vi "PQexecuteCommand.vi"(0 "conn":u64, 5 "Command":string, 11 "error in (no error)":errorcluster) -> (4 "conn_out":u64, 6 "Data":string[][](array[string]), 8 "ColumnNames":string[](array[string]), 10 "ColsCount":i64, 13 "error out":errorcluster, 14 "DatabaseMesssageCluster":T1, 15 "RowsCount":i64)   [LabVIEW 2019, in "libpqutility64.lvlib"]
doc: "Send arbitrari SQL command against PostgreSQL database, and fetch the result data into string array.\nSee PostgreSQL c-lib doku for further information."
uses:
  libpqutility64.lvlib
  libpqlv64/libpqlv64.lvlib
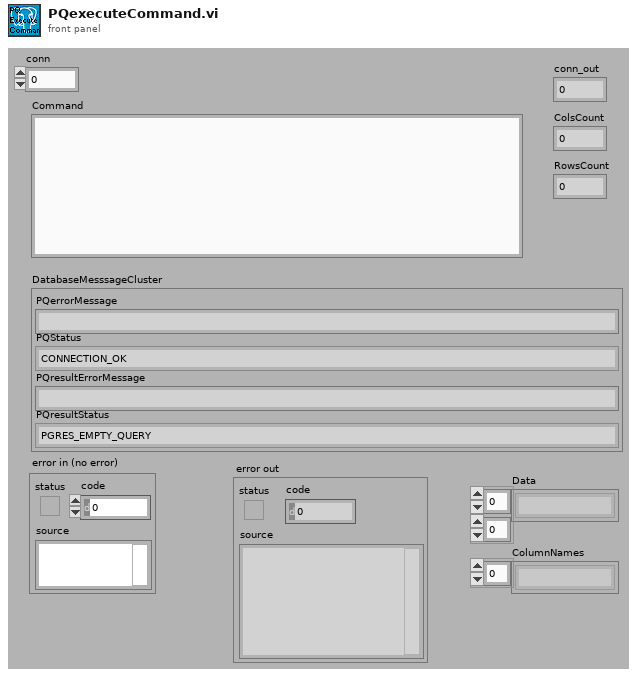
[diagram p1: front panel]
types:
  T1 = cluster{"PQerrorMessage":string, "PQStatus":enum16{"CONNECTION_OK", "CONNECTION_BAD", "CONNECTION_STARTED", "CONNECTION_MADE", "CONNECTION_AWAITING_RESPONSE", "CONNECTION_AUTH_OK", "CONNECTION_SETENV", "CONNECTION_SSL_STARTUP", "CONNECTION_NEEDED"}, "PQresultErrorMessage":string, "PQresultStatus":enum16{"PGRES_EMPTY_QUERY", "PGRES_COMMAND_OK", "PGRES_TUPLES_OK", "PGRES_COPY_OUT", "PGRES_COPY_IN", "PGRES_BAD_RESPONSE", "PGRES_NONFATAL_ERROR", "PGRES_FATAL_ERROR"}}
  T2 = enum16{"PGRES_EMPTY_QUERY", "PGRES_COMMAND_OK", "PGRES_TUPLES_OK", "PGRES_COPY_OUT", "PGRES_COPY_IN", "PGRES_BAD_RESPONSE", "PGRES_NONFATAL_ERROR", "PGRES_FATAL_ERROR"}
  T3 = enum32{"PGRES_EMPTY_QUERY", "PGRES_COMMAND_OK", "PGRES_TUPLES_OK", "PGRES_COPY_OUT", "PGRES_COPY_IN", "PGRES_BAD_RESPONSE", "PGRES_NONFATAL_ERROR", "PGRES_FATAL_ERROR"}
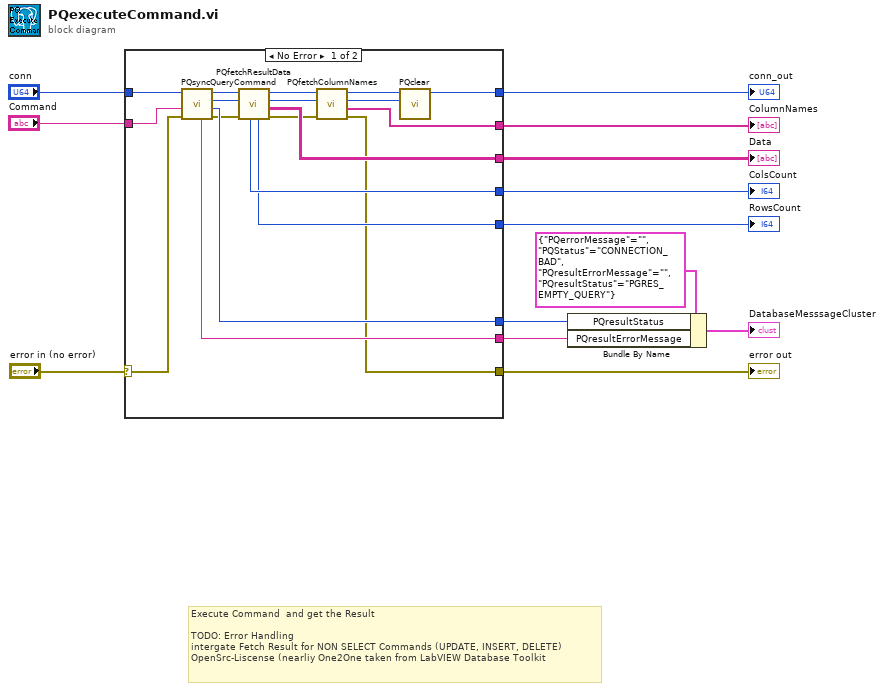
[diagram p0: block diagram]
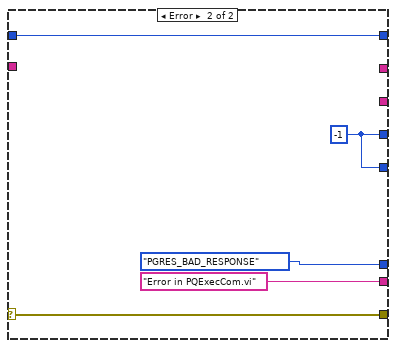
[diagram p2: hidden frame]
diagram:
  # "Execute Command  and get the Result\n\nTODO: Error Handling\nintergate Fetch Result for NON SELECT Commands (UPDATE, INSERT, DELETE)\nOpenSrc-Liscense (nearliy One2One taken from LabVIEW Database Toolkit"
  n1 = case shown="No Error" "error in (no error)" {
    selector: "error in (no error)" -> [w17 w33]
    tunnel: [w14 w33] -> w9
    tunnel: "conn" -> [w32 w37]
    tunnel: [w28 _] -> w13
    tunnel: [w29 w37] -> w2
    tunnel: [w23 _] -> w12
    tunnel: [w22 w36] -> w11
    tunnel: [w21 w36] -> w10
    tunnel: "Command" -> [w20 _]
    tunnel: [w19 T2."PGRES_BAD_RESPONSE" ("PQresultStatus")] -> w6
    tunnel: [w18 "Error in PQExecCom.vi" ("PQresultErrorMessage")] -> w5
    frame No Error {
      n2 = call "PQsyncQueryCommand.vi"("error in (no error)"=w17, "query"=w20, "conn"=w32) -> ("error out"=w16:errorcluster, "PQresultStatus"=w19:T3, "PGresult"=w31:u64, "conn out"=w30:u64, "PQresultErrorMessage"=w18:string)  [unwired: 4 in]
      n3 = call "PQfetchResultData.vi"("error in"=w16, "res"=w31, "conn"=w30) -> ("error out"=w15:errorcluster, "Data"=w28:string[][], "res_out"=w27:u64, "conn_out"=w26:u64, "PQnFields"=w21:i64, "PQnTuples"=w22:i64)  [unwired: 3 in]
      n4 = call "PQfetchColumnNames.vi"("error in"=w15, "res"=w27, "conn"=w26) -> ("error out"=w14:errorcluster, "ColumnNames"=w23:string[], "res_out"=w24:u64, "conn_out"=w25:u64)  [unwired: 3 in]
      n5 = call "PQclear.vi"("res"=w24, "conn"=w25) -> ("conn_out"=w29:u64)  [unwired: 8 in, 1 out]
    }
    frame Error {
      w36 = i64 -1 ("PQnFields")
    }
  }
  "error out" <- w9
  "Data" <- w13
  "conn_out" <- w2
  "ColumnNames" <- w12
  "ColsCount" <- w11
  "RowsCount" <- w10
  n6 = Bundle By Name(cluster=T1 {"PQerrorMessage"="", "PQStatus"=enum."CONNECTION_BAD", "PQresultErrorMessage"="", "PQresultStatus"=enum."PGRES_EMPTY_QUERY"} ("Database Status Message 2"), "PQresultStatus"=w6, "PQresultErrorMessage"=w5) -> (→"DatabaseMesssageCluster":T1)
